vi "Analog Input Voltages.vi"(8 "error in (no error)":errorcluster, 10 "Analog Input Voltages":waveform(dbl)[](array[waveform]), 11 "Top in":refnum<class "Top.lvclass">) -> (0 "error out":errorcluster, 3 "Top out":refnum<class "Top.lvclass">)   [LabVIEW 2021, in "Top.lvlib" / "Top.lvclass"]
uses:
  Top.lvclass
  Top.lvclass/Top.ctl
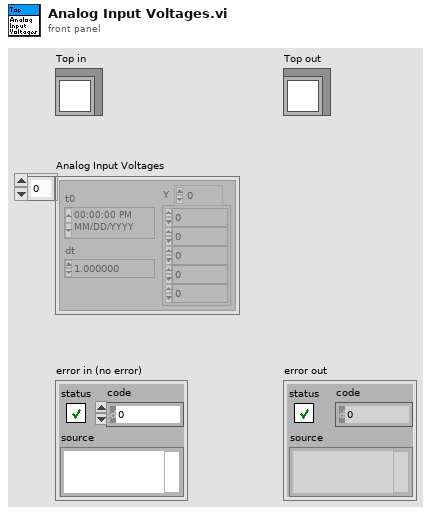
[diagram p1: front panel]
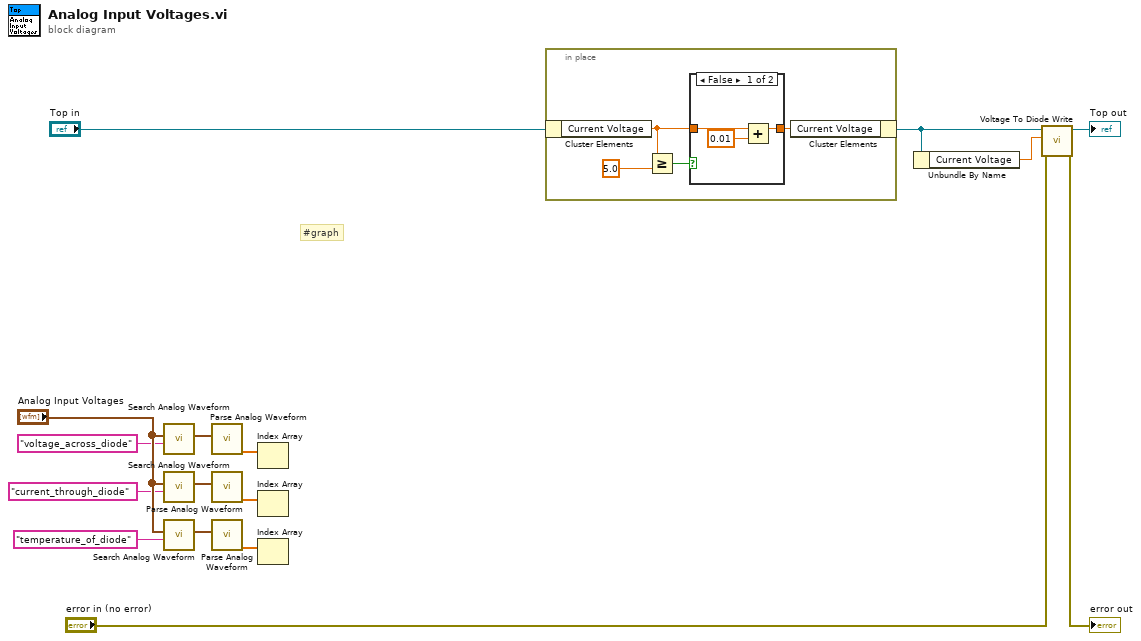
[diagram p0: block diagram]
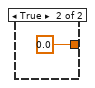
[diagram p2: hidden frame]
diagram:
  # "#graph"
  n1 = call <vilib>:"Search Analog Waveform.vi"("NI_ChannelName"="voltage_across_diode", "Waveforms"="Analog Input Voltages") -> ("Waveform"=w15:waveform(dbl))  [unwired: 8 in, 1 out]
  n2 = call <vilib>:"Search Analog Waveform.vi"("NI_ChannelName"="current_through_diode", "Waveforms"="Analog Input Voltages") -> ("Waveform"=w14:waveform(dbl))  [unwired: 8 in, 1 out]
  n3 = call <vilib>:"Search Analog Waveform.vi"("NI_ChannelName"="temperature_of_diode", "Waveforms"="Analog Input Voltages") -> ("Waveform"=w13:waveform(dbl))  [unwired: 8 in, 1 out]
  n4 = call <vilib>:"Parse Analog Waveform.vi"("Waveform"=w15) -> ("Y"=w1:dbl[])  [unwired: 7 in, 3 out]
  n5 = call <vilib>:"Parse Analog Waveform.vi"("Waveform"=w14) -> ("Y"=w2:dbl[])  [unwired: 7 in, 3 out]
  n6 = call <vilib>:"Parse Analog Waveform.vi"("Waveform"=w13) -> ("Y"=w3:dbl[])  [unwired: 7 in, 3 out]
  n7 = Index Array(array=w1) -> ()  [unwired: 1 in, 1 out]
  n8 = Index Array(array=w2) -> ()  [unwired: 1 in, 1 out]
  n9 = Index Array(array=w3) -> ()  [unwired: 1 in, 1 out]
  n10 = in-place {
    n11 = in-place-cluster #1("Top in") -> ("Current Voltage"=w18:dbl)
    n12 = Greater Or Equal?(x=w18, y=5.0) -> (x >= y?=w20:bool)
    n13 = case shown="False" w20 {
      tunnel: w18 -> [w23 _]
      tunnel: [w22 0.0] -> w19
      frame False {
        n14 = Add(x=w23, y=0.01) -> (x+y=w22:dbl)
      }
      frame True {
      }
    }
    n15 = in-place-cluster #1("Current Voltage"=w19) -> (w5:refnum<class "Top.lvclass">)
  }
  n16 = Unbundle By Name(w5) -> ("Current Voltage"=w4:dbl)
  n17 = call "Voltage To Diode Write.vi"("error in (no error)"="error in (no error)", "Voltage"=w4, "Top in"=w5) -> ("error out"=→"error out":errorcluster, "Top out"=→"Top out":refnum<class "Top.lvclass">)  [unwired: 7 in]
